vi "Get Model.vi"(8 "error in (no error)":errorcluster, 11 "Device in":refnum<class "Device.lvclass">) -> (0 "error out":errorcluster, 2 "Model":string, 3 "Device out":refnum<class "Device.lvclass">)   [LabVIEW 2012, in "HAL.lvlib" / "Device.lvclass"]
doc: "Concrete device classes need to override this VI to provide the string value that uniquely identifies a device's capabilities such as Keithley 2300. Any devices that provide the same methods and have the same communication channel can all use the same concrete device type."
uses:
  Device.lvclass
  <vilib>/Utility/error.llb/Error Cluster From Error Code.vi
  <vilib>/ErrorRing/Error Ring.xnode
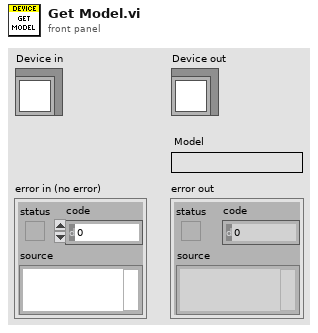
[diagram p1: front panel]
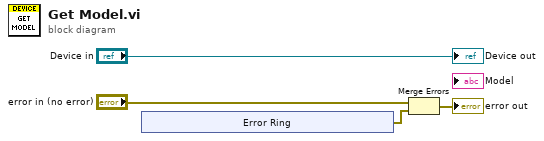
[diagram p0: block diagram]
diagram:
  n1 = xnode "Error Ring"() -> ("error out"=w3:errorcluster)
  n2 = Merge Errors("error in (no error)", w3) -> (→"error out":errorcluster)
  "Device out" <- "Device in"
